vi "FGV_ARCH_EDITOR_records_display.vi"(4 "front_panel_reference":refnum<vi>, 6 "SQL_listbox_reference":refnum<vi>, 7 "options":T3, 8 "error_in":errorcluster, 10 "uneditable_columns":string[](array[string])=["ID", "CREATION_TIME", "CREATED_BY"], 11 "input":variant) -> (0 "error_out":errorcluster, 1 "all_info":T1, 2 "array_param_output":string[](array[string]), 3 "string_param_output":string)   [LabVIEW 2019]
uses:
  FGV_ARCH_EDITOR_records_display.ctl
  ARCH_EDITOR_all_info.ctl
  MAIN/SQL_record_states.ctl
  ini/typedef/CLIENT_all_config_info.ctl
  ini/typedef/CLIENT_main_ini_file.ctl
  queues/typedef/CLIENT_queue_refnums.ctl
  queues/typedef/SQL_EDITOR_queue_element.ctl
  MAIN/SQL_EDITOR/SQL_EDITOR_sequence_state.ctl
  queues/typedef/CLIENT_SCANNER_queue_element.ctl
  MAIN/SCANNER/SCANNER_sequence_state.ctl
  queues/typedef/CLIENT_REF_CHG_queue_element.ctl
  MAIN/reference_changed_connection/CLIENT_REF_CHG_sequence_state.ctl
  login/FGV_login.ctl
  <userlib>/_OpenG.lib/array/array.llb/Filter 1D Array (String)__ogtk.vi
  <userlib>/_OpenG.lib/array/array.llb/Delete Elements from 1D Array (I32)__ogtk.vi
  <vilib>/addons/database/_DB Variant To Data/Database Variant To Data.xnode
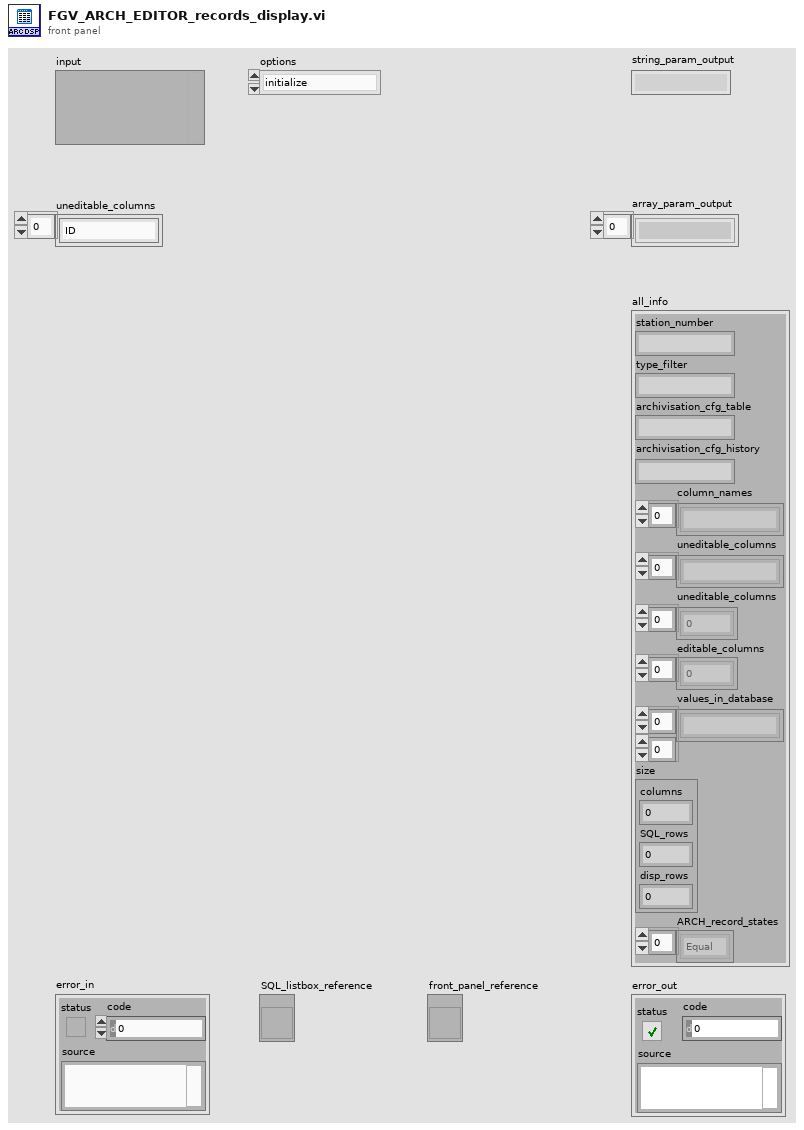
[diagram p1: front panel]
types:
  T1 = typedef "ARCH_EDITOR_all_info.ctl" = cluster{"station_number":string, "type_filter":string, "archivisation_cfg_table":string, "archivisation_cfg_history":string, "column_names":string[], "uneditable_columns":string[], "uneditable_columns":i32[], "editable_columns":i32[], "values_in_database":string[][], "size":cluster{"columns":i32, "SQL_rows":i32, "disp_rows":i32}, "ARCH_record_states":T2[]}
  T2 = typedef "SQL_record_states.ctl" = enum16{"Equal", "Added", "Edited", "Deleted"}
  T3 = typedef "FGV_ARCH_EDITOR_records_display.ctl" = enum16{"initialize", "set_arch_cfg_tables_names", "set_station_number", "set_type_filter", "set_headers", "set_records", "get_arch_cfg_table_name", "get_arch_cfg_hist_table_name", "get_station_number", "get_type_filter", "get_headers", "get_uneditable_columns", "get_all_info", "record_added?", "record_inserted?", "record_edited?", "record_updated?", "record_deleted?", "discard_changes"}
  T4 = typedef "CLIENT_all_config_info.ctl" = cluster{"main_ini_file":T5, "SQL Password":string, "queue_refnums":T6}
  T5 = typedef "CLIENT_main_ini_file.ctl" = cluster{"SQL Driver":string, "SQL Server":string, "SQL Database":string, "SQL UID":string, "Reference table":string, "Reference history":string, "Archivisation CFG table":string, "Archivisation CFG history":string, "User table":string, "User history":string, "logout timeout [ms]":i32, "records per page":i32, "default language":string, "REF CHG connection IP":string, "REF CHG remote port":i32, "REF CHG local port":i32, "SCANNER COM port":u16, "SCANNER Baud rate":u32, "SCANNER Data bits":u16, "SCANNER Pairity":enum16{"None", "Odd", "Even", "Mark", "Space"}, "SCANNER Stop bits":u16, "SCANNER Flow control":u16, "SCANNER Termination char":u8}
  T6 = typedef "CLIENT_queue_refnums.ctl" = cluster{"SQL_EDITOR_queue":refnum<queue>, "SCANNER_queue":refnum<queue>, "SCANNER_data":refnum<queue>, "CLIENT_REF_CHG_queue":refnum<queue>}
  T7 = typedef "FGV_login.ctl" = enum16{"initialize", "login", "logout", "get_login_info"}
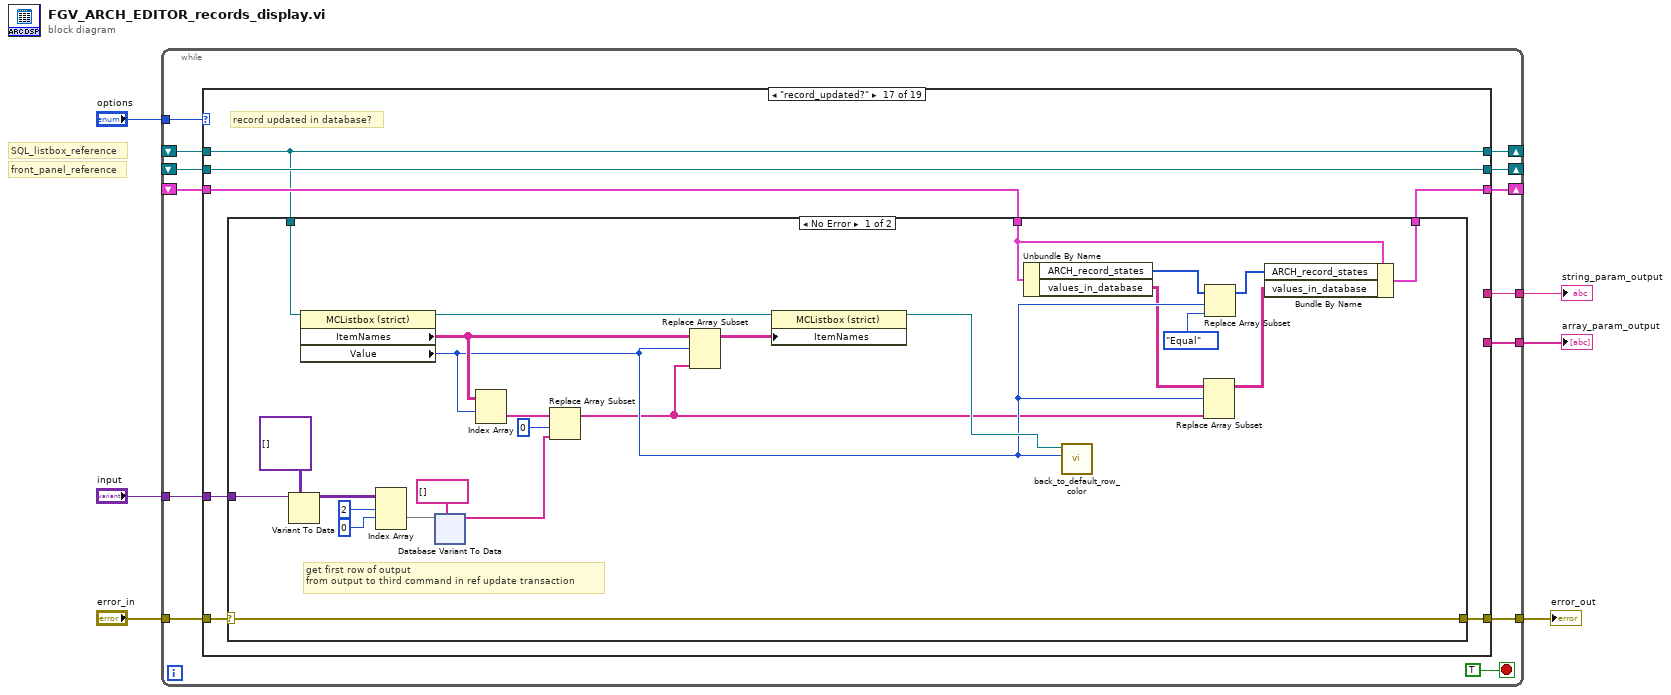
[diagram p0: block diagram]
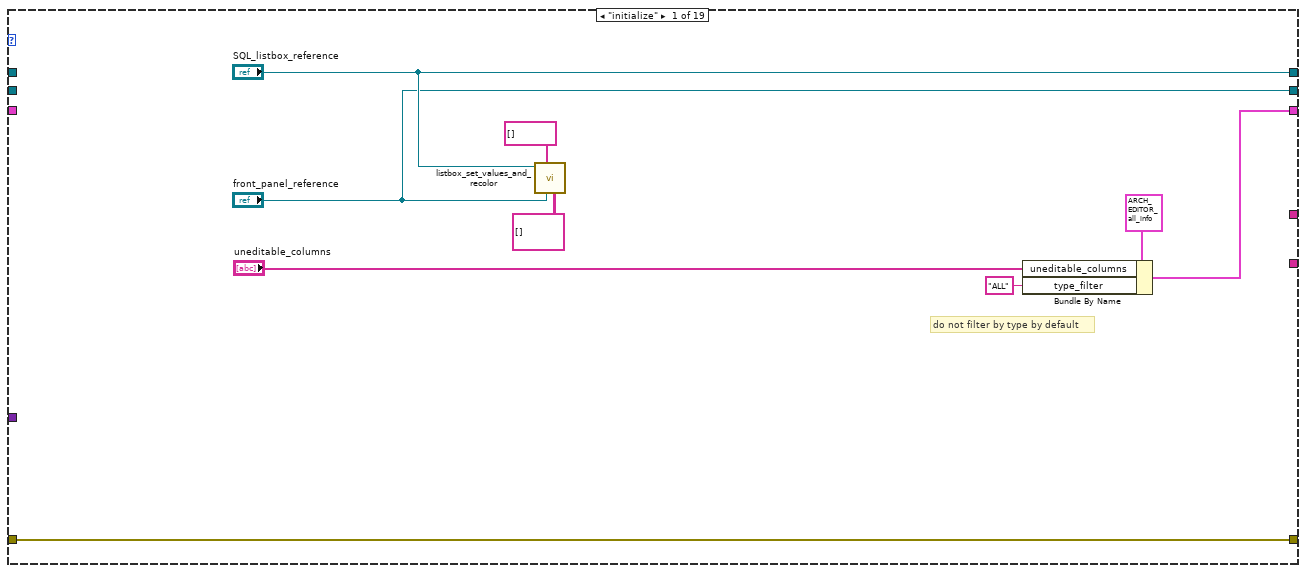
[diagram p2: hidden frame]
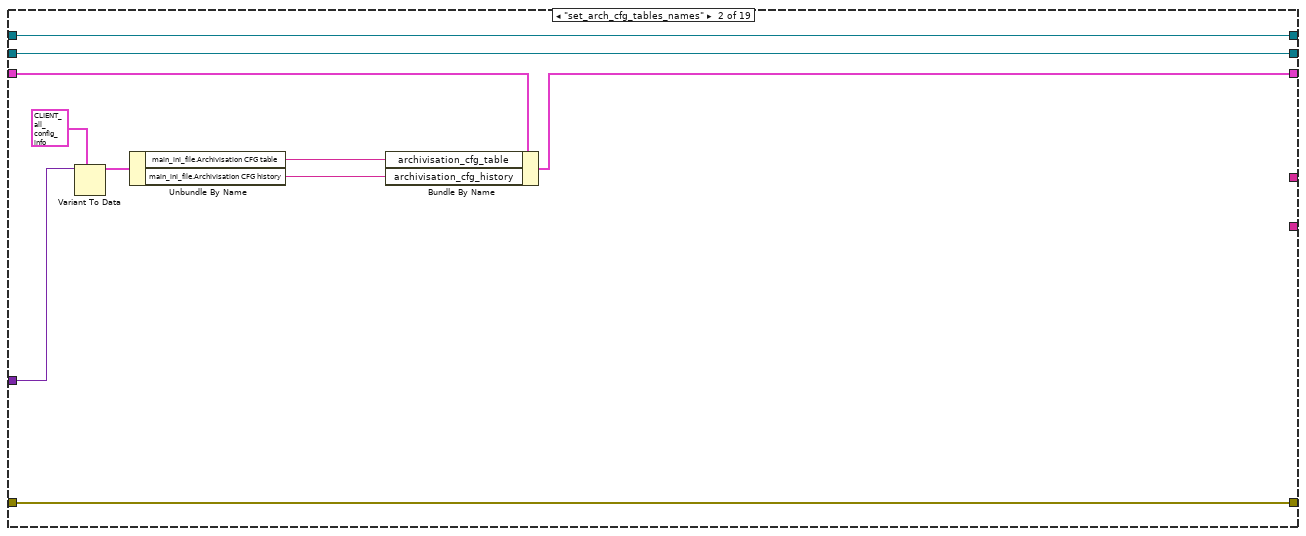
[diagram p3: hidden frame]
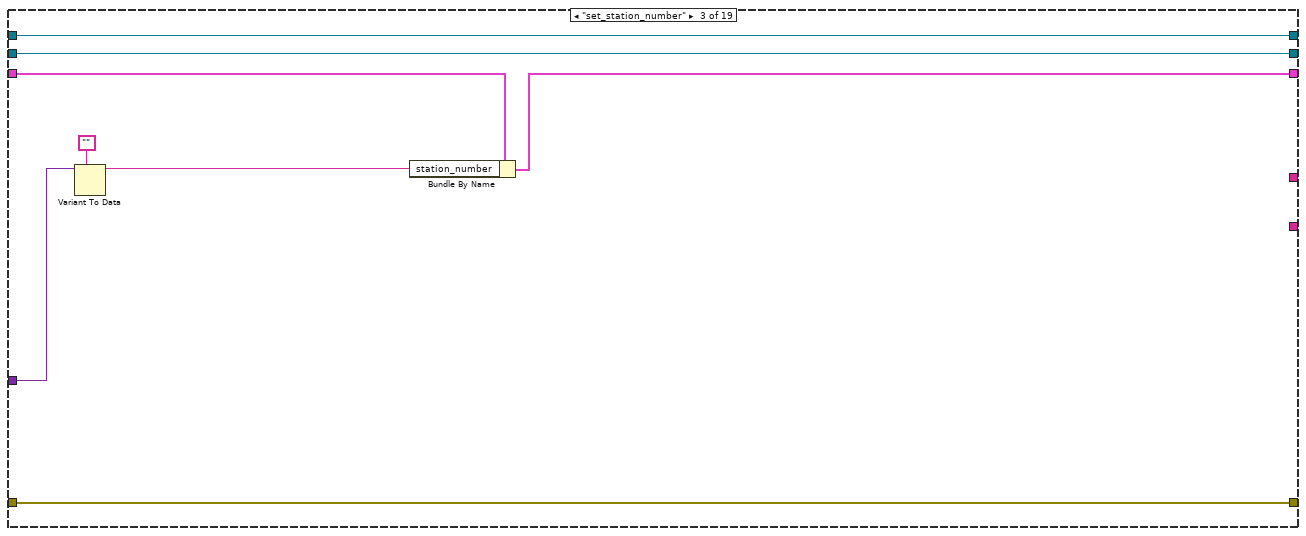
[diagram p4: hidden frame]
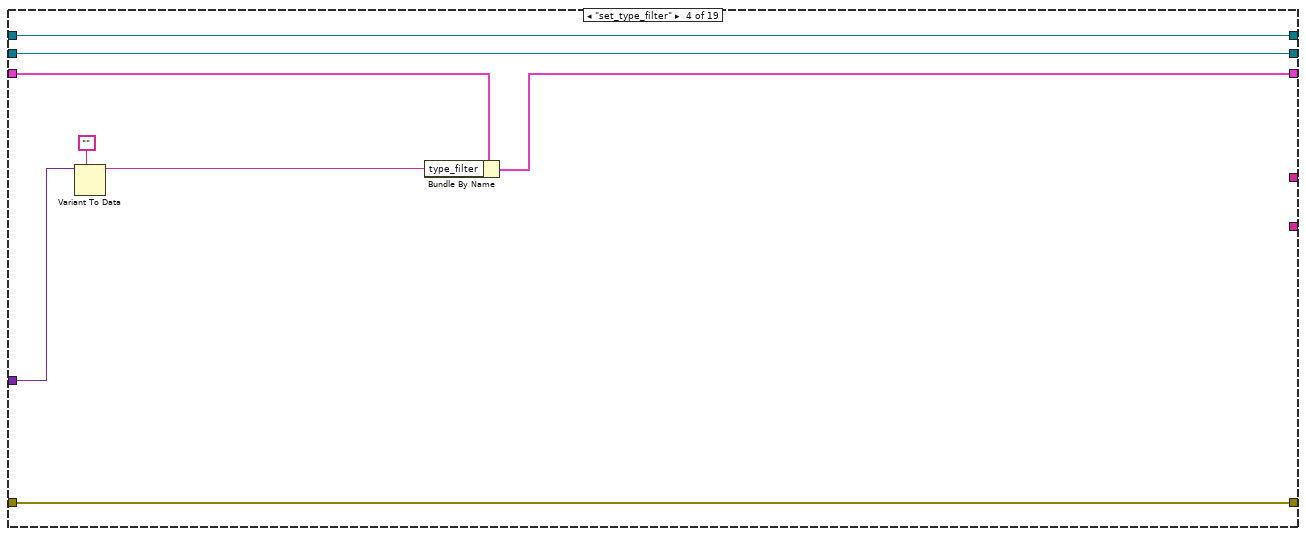
[diagram p5: hidden frame]
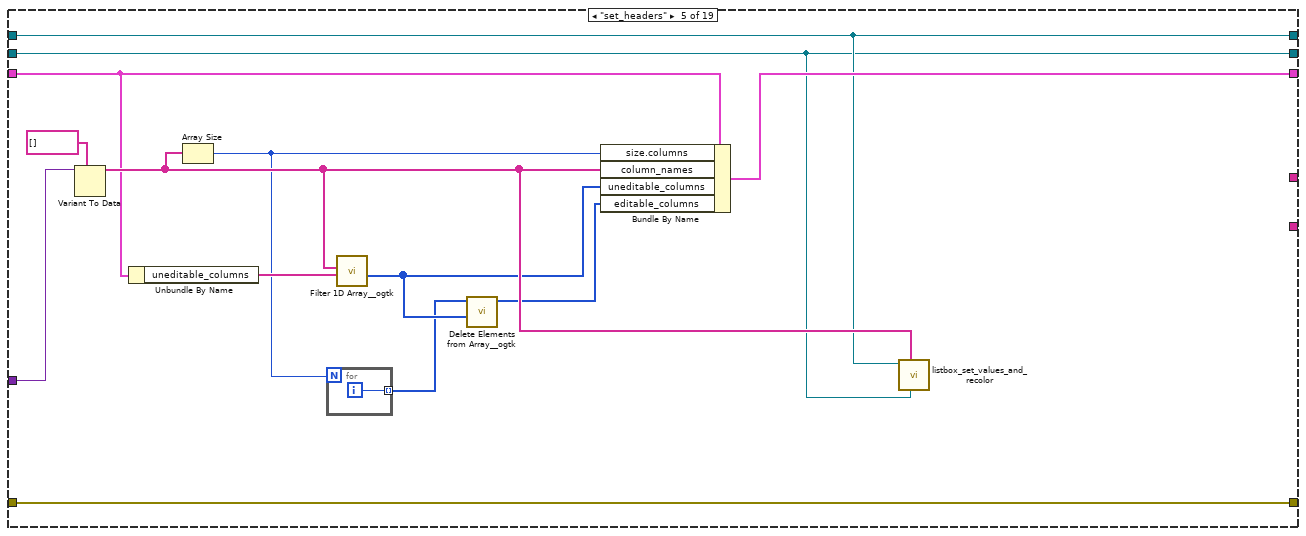
[diagram p6: hidden frame]
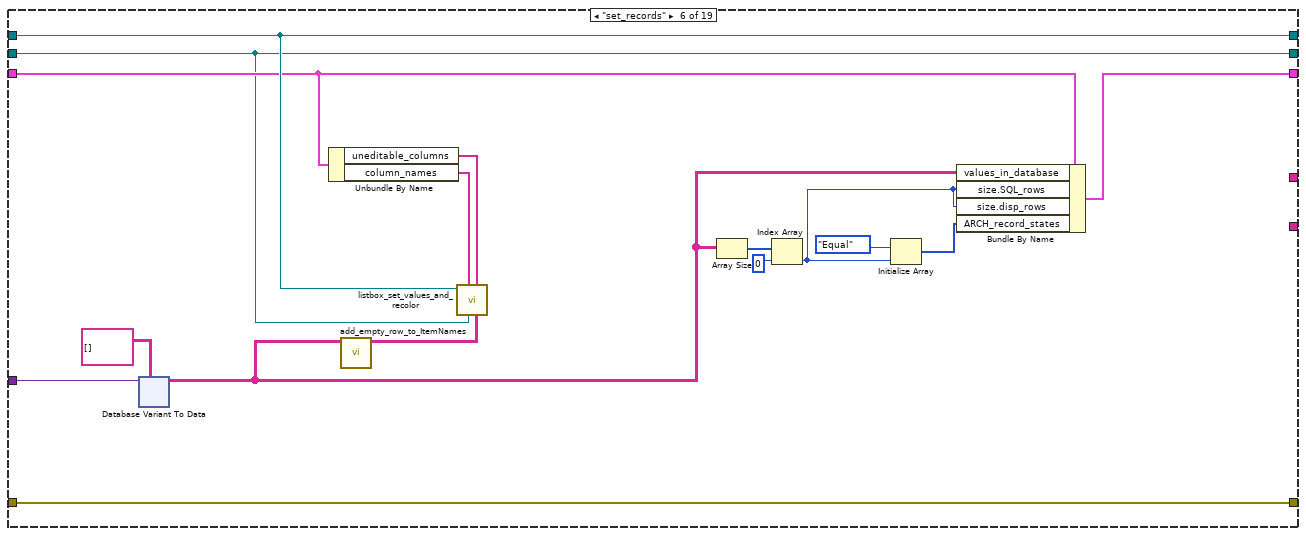
[diagram p7: hidden frame]
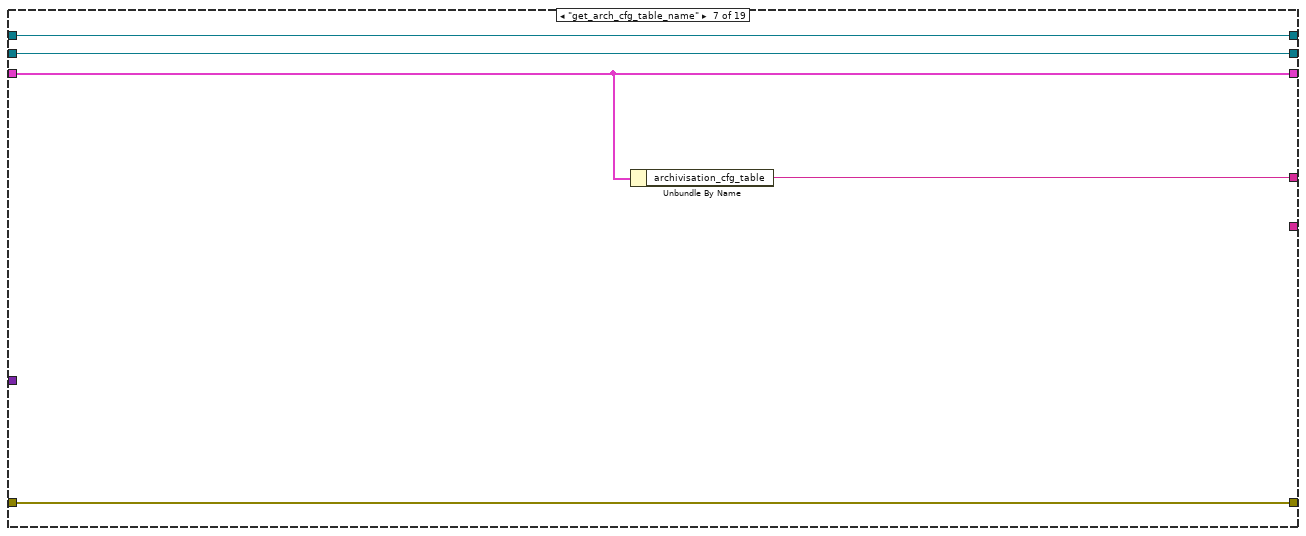
[diagram p8: hidden frame]
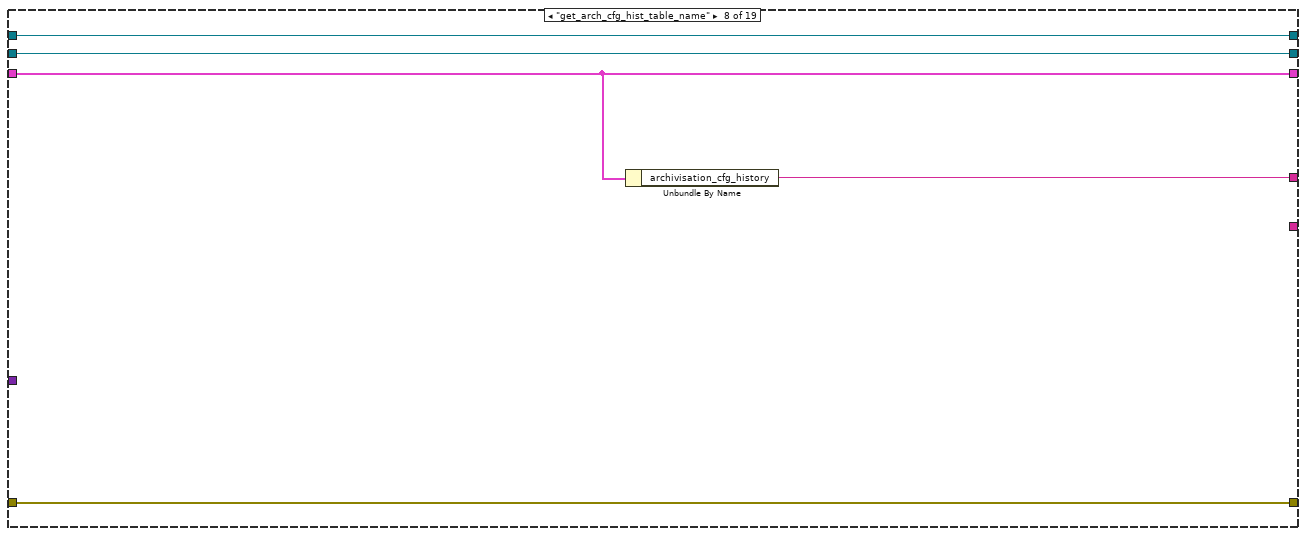
[diagram p9: hidden frame]
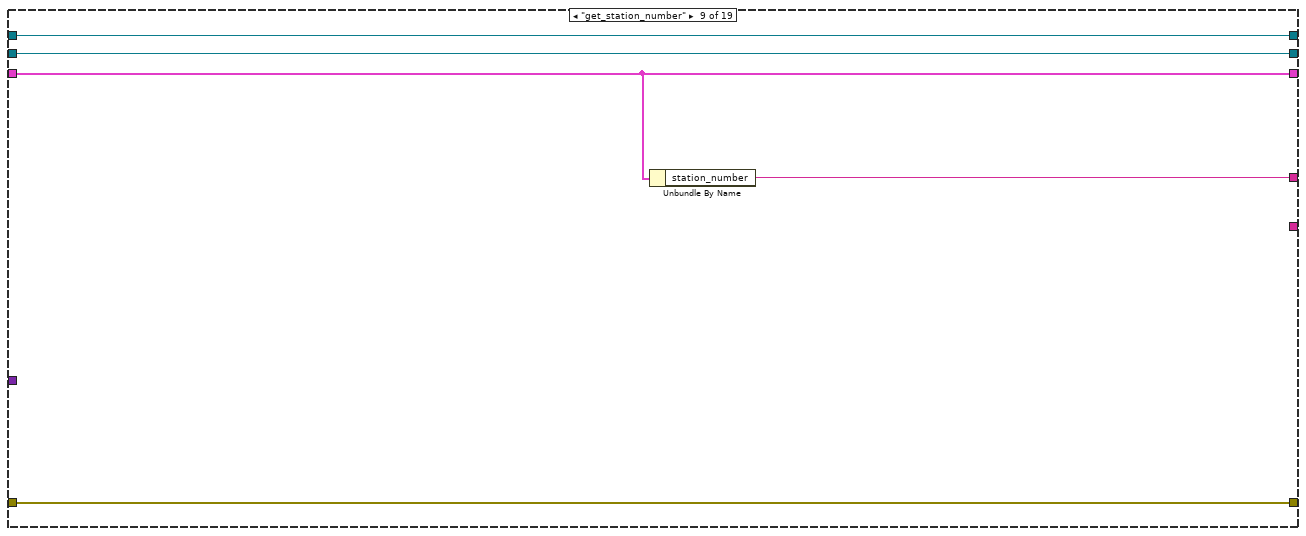
[diagram p10: hidden frame]
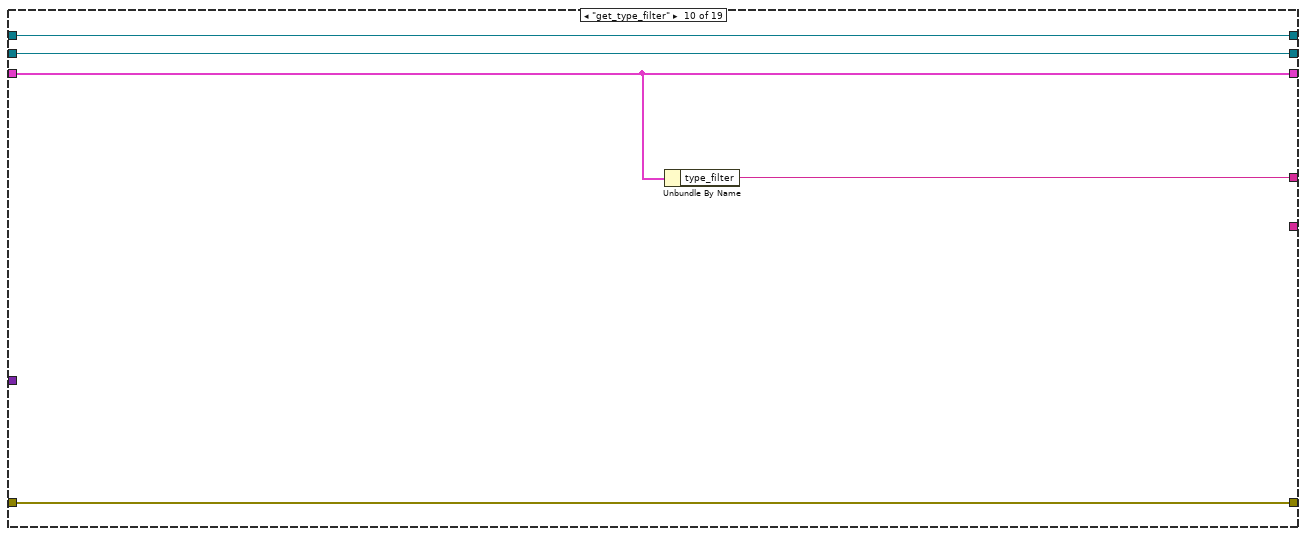
[diagram p11: hidden frame]
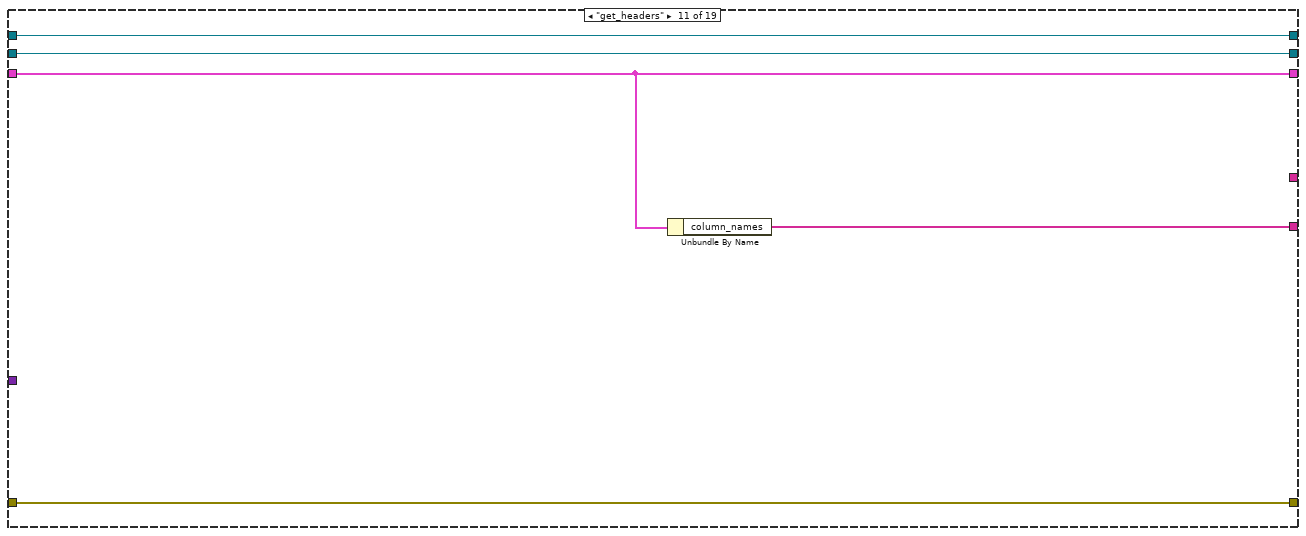
[diagram p12: hidden frame]
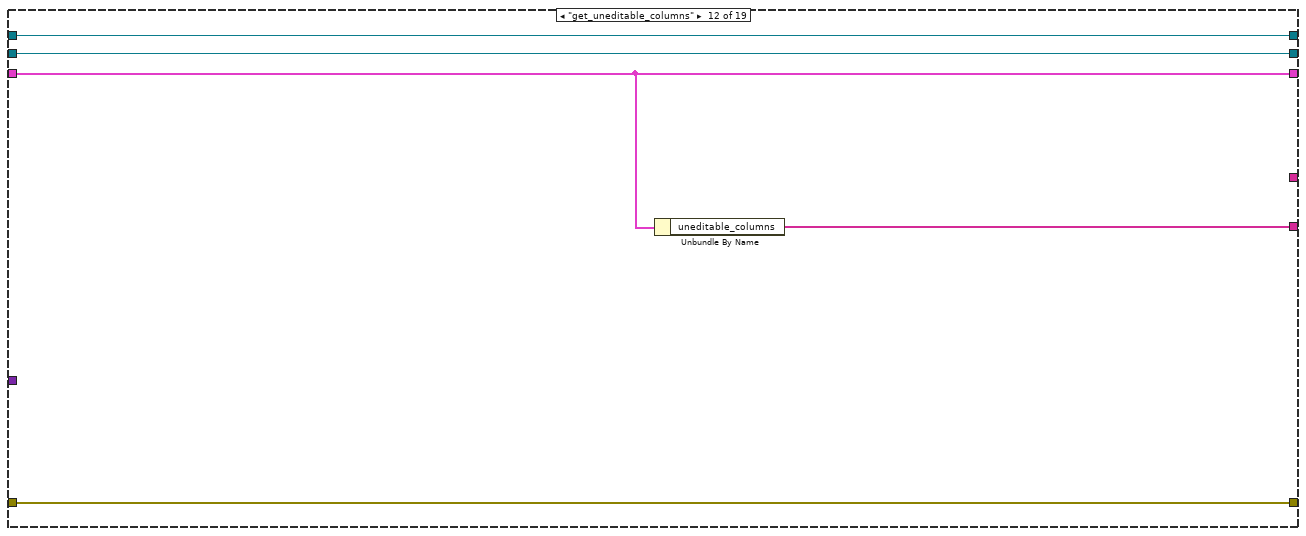
[diagram p13: hidden frame]
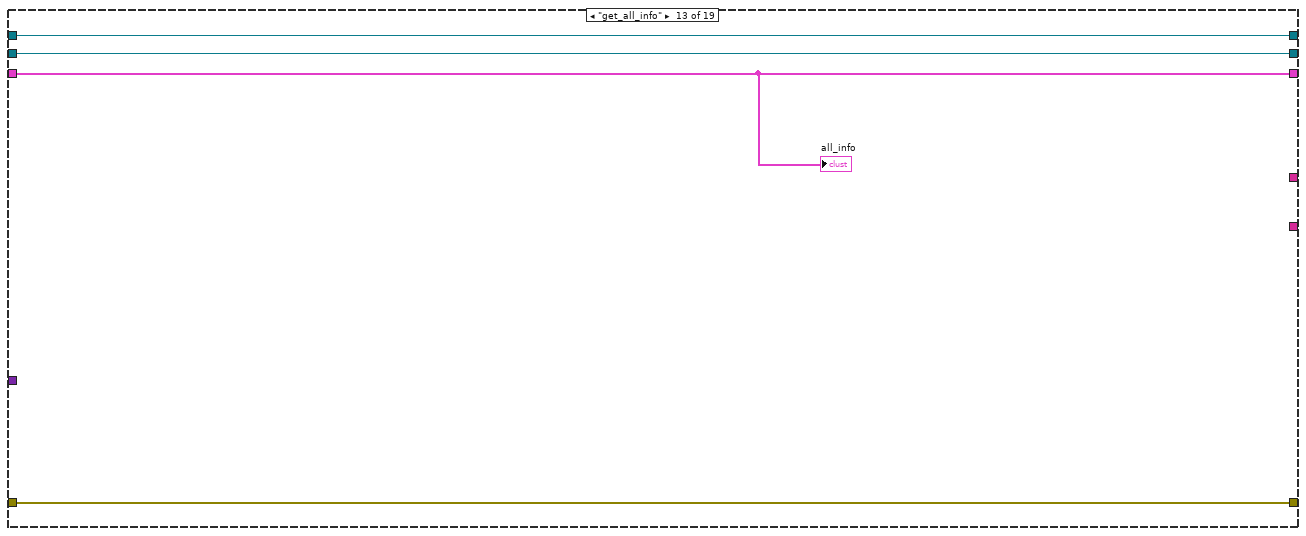
[diagram p14: hidden frame]
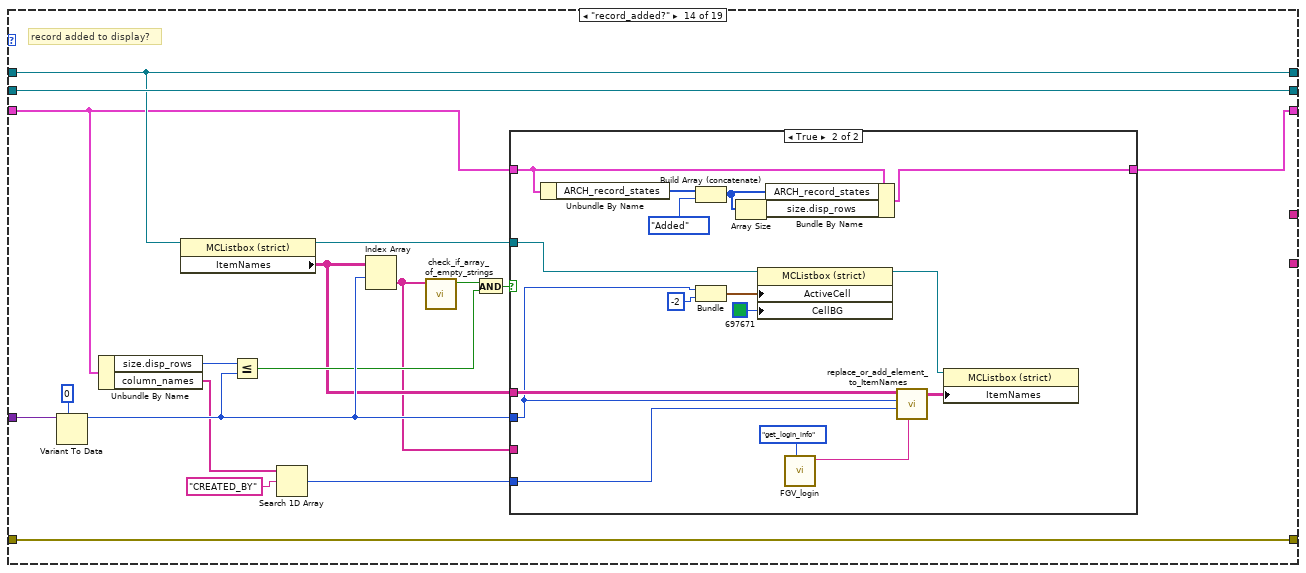
[diagram p15: hidden frame]
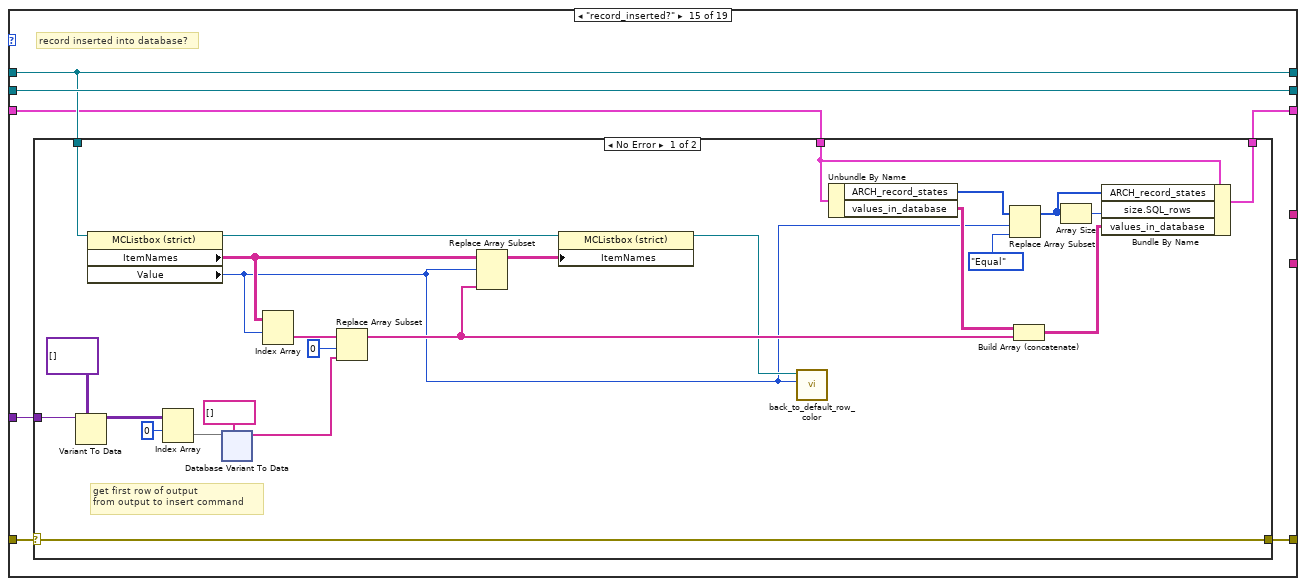
[diagram p17: hidden frame]
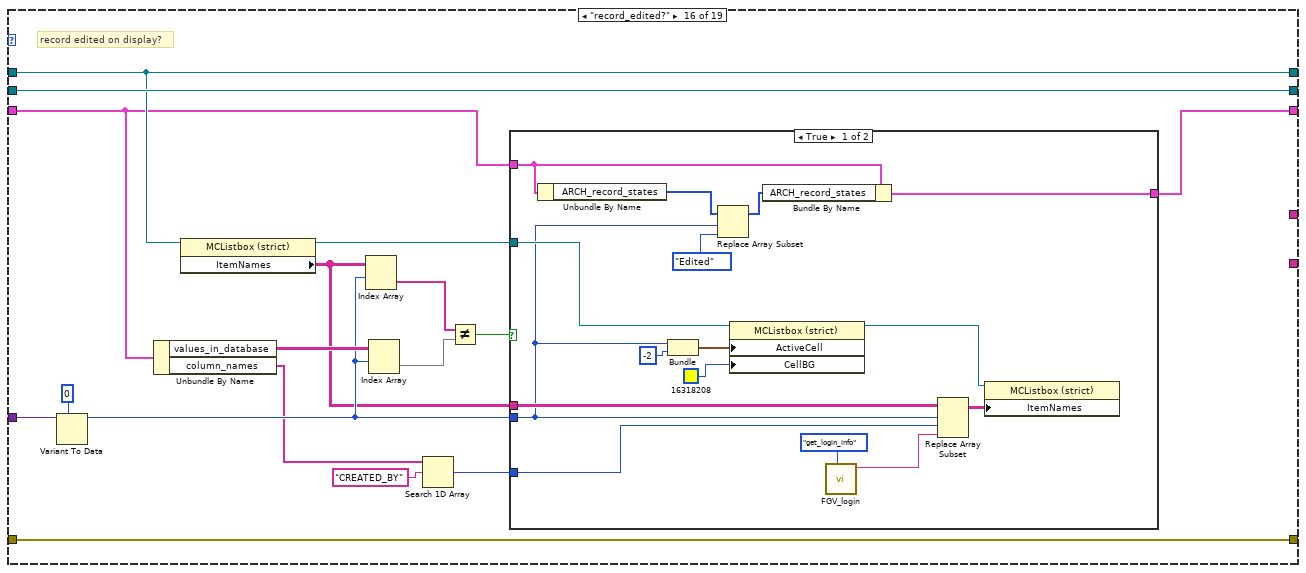
[diagram p19: hidden frame]
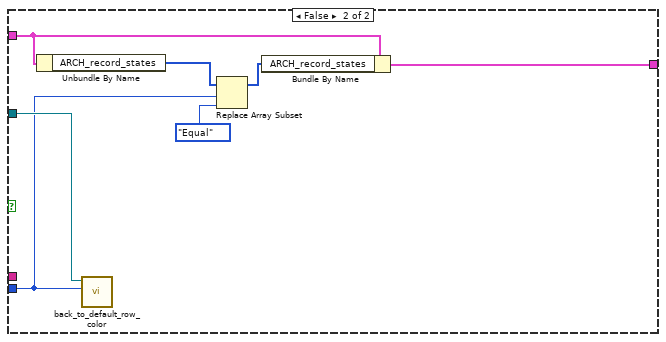
[diagram p20: hidden frame]
diagram:
  # "front_panel_reference"
  # "SQL_listbox_reference"
  n1 = while {
    tunnel: "options" -> [w18]
    tunnel: [w17] -> w6
    tunnel: "error_in" -> [w16]
    shift-right: [w15] -> _
    shift-left: _ -> [w14]
    tunnel: [w13] -> w3
    shift-right: [w12] -> _
    shift-left: _ -> [w11]
    tunnel: [w10] -> w2
    tunnel: "input" -> [w9]
    shift-right: [w8] -> _
    shift-left: _ -> [w7]
    stop <- TRUE stop-if-true
    n2 = case shown="\"record_updated?\"" w18 {
      tunnel: [w28 w38 w46 w54 w67 w82 w119 w124 w129 w134 w140 w145 w149 w168 w192 w275 w304 w372 w397] -> w17
      tunnel: w16 -> [w28 w38 w46 w54 w67 w82 w119 w124 w129 w134 w140 w145 w149 w168 w191 w275 w303 w373 w397]
      tunnel: [w24 w36 w44 w52 w57 w78 w121 w126 w131 w136 w141 w146 w150 w162 w188 w263 w300 w374 w398] -> w15
      tunnel: w14 -> [_ w37 w45 w53 w58 w79 w121 w126 w131 w136 w141 w146 w150 w161 w189 w264 w301 w375 w393]
      tunnel: [_ _ _ _ _ _ w120 w125 w130 w135 _ _ _ _ _ _ _ _ _] -> w13
      tunnel: ["SQL_listbox_reference" w35 w43 w51 w56 w81 w118 w123 w128 w133 w137 w144 w148 w164 w190 w270 w299 w377 w392] -> w12
      tunnel: w11 -> [_ w35 w43 w51 w56 w81 w118 w123 w128 w133 w137 w144 w148 w164 w190 w270 w299 w377 w392]
      tunnel: [_ _ _ _ _ _ _ _ _ _ w139 w143 _ _ _ _ _ _ _] -> w10
      tunnel: w9 -> [_ w34 w42 w50 w59 w83 _ _ _ _ _ _ _ w166 w187 w273 w302 _ _]
      tunnel: ["front_panel_reference" w33 w39 w47 w55 w71 w117 w122 w127 w132 w138 w142 w147 w167 w193 w274 w305 w378 w400] -> w8
      tunnel: w7 -> [_ w33 w39 w47 w55 w71 w117 w122 w127 w132 w138 w142 w147 w167 w193 w274 w305 w378 w400]
      frame "initialize" {
        # "do not filter by type by default"
        n3 = call "listbox_set_values_and_recolor.vi"("item_names"=string[][] [], "front_panel_reference"="front_panel_reference", "column_names"=string[] [], "multicolumn_listbox_reference_in"="SQL_listbox_reference") -> ()  [unwired: 6 in, 2 out]
        n4 = Bundle By Name(cluster=T1 {"station_number"="", "type_filter"="", "archivisation_cfg_table"="", "archivisation_cfg_history"="", "column_names"=[], "uneditable_columns"=[], "uneditable_columns"=[], "editable_columns"=[], "values_in_database"=[], "size"={"columns"=0, "SQL_rows"=0, "disp_rows"=0}, "ARCH_record_states"=[]} ("SQL_selection"), "uneditable_columns"="uneditable_columns", "type_filter"="ALL") -> (w24:T1)
      }
      frame "set_arch_cfg_tables_names" {
        n5 = Variant To Data(type=T4 {"main_ini_file"={"SQL Driver"="", "SQL Server"="", "SQL Database"="", "SQL UID"="", "Reference table"="", "Reference history"="", "Archivisation CFG table"="", "Archivisation CFG history"="", "User table"="", "User history"="", "logout timeout [ms]"=0, "records per page"=0, "default language"="", "REF CHG connection IP"="", "REF CHG remote port"=0, "REF CHG local port"=0, "SCANNER COM port"=0, "SCANNER Baud rate"=0, "SCANNER Data bits"=0, "SCANNER Pairity"=enum."None", "SCANNER Stop bits"=10, "SCANNER Flow control"=0, "SCANNER Termination char"=0}, "SQL Password"="", "queue_refnums"={"SQL_EDITOR_queue"=refnum, "SCANNER_queue"=refnum, "SCANNER_data"=refnum, "CLIENT_REF_CHG_queue"=refnum}} ("all_config_info"), Variant=w34) -> (data=w32:T4)  [unwired: 1 in, 1 out]
        n6 = Unbundle By Name(w32) -> ("main_ini_file.Archivisation CFG table"=w31:string, "main_ini_file.Archivisation CFG history"=w30:string)
        n7 = Bundle By Name(cluster=w37, "archivisation_cfg_table"=w31, "archivisation_cfg_history"=w30) -> (w36:T1)
      }
      frame "set_station_number" {
        n8 = Variant To Data(type="", Variant=w42) -> (data=w40:string)  [unwired: 1 in, 1 out]
        n9 = Bundle By Name(cluster=w45, "station_number"=w40) -> (w44:T1)
      }
      frame "set_type_filter" {
        n10 = Variant To Data(type="", Variant=w50) -> (data=w48:string)  [unwired: 1 in, 1 out]
        n11 = Bundle By Name(cluster=w53, "type_filter"=w48) -> (w52:T1)
      }
      frame "set_headers" {
        n12 = Variant To Data(type=string[] [], Variant=w59) -> (data=w65:string[])  [unwired: 1 in, 1 out]
        n13 = Unbundle By Name(w58) -> ("uneditable_columns"=w63:string[])
        n14 = Array Size(array=w65) -> (size(s)=w60:i32)
        n15 = for {
          N: w60 -> [_]
          tunnel: [w68] -> w62 mode=indexing
          i -> [w68]
        }
        n16 = call-poly <userlib>:"Filter 1D Array__ogtk.vi"("items to filter"=w63, "array"=w65) -> ("filtered item indices"=w64:i32[])  [unwired: 4 in, 1 out]
        n17 = call-poly <userlib>:"Delete Elements from Array__ogtk.vi"("indices"=w64, "array"=w62) -> ("array w/ subset deleted"=w61:i32[])  [unwired: 8 in, 1 out]
        n18 = Bundle By Name(cluster=w58, "size.columns"=w60, "column_names"=w65, "uneditable_columns"=w64, "editable_columns"=w61) -> (w57:T1)
        n19 = call "listbox_set_values_and_recolor.vi"("front_panel_reference"=w55, "column_names"=w65, "multicolumn_listbox_reference_in"=w56) -> ()  [unwired: 7 in, 2 out]
      }
      frame "set_records" {
        n20 = xnode "Database Variant To Data"("database variant"=w83, "type"=string[][] []) -> ("data"=w69:string[][])  [unwired: 1 in, 1 out]
        n21 = Unbundle By Name(w79) -> ("uneditable_columns"=w72:string[], "column_names"=w80:string[])
        n22 = call "add_empty_row_to_ItemNames.vi"("ItemNames_in"=w69) -> ("ItemNames_out"=w70:string[][])  [unwired: 10 in]
        n23 = call "listbox_set_values_and_recolor.vi"("item_names"=w70, "uneditable_columns"=w72, "front_panel_reference"=w71, "column_names"=w80, "multicolumn_listbox_reference_in"=w81) -> ()  [unwired: 5 in, 2 out]
        n24 = Array Size(array=w69) -> (size(s)=w77:i32[])
        n25 = Index Array(array=w77, index=0) -> (element=w74:i32)
        n26 = Initialize Array(SQL_record_states."Equal", w74) -> (w73:T2[])
        n27 = Bundle By Name(cluster=w79, "values_in_database"=w69, "size.SQL_rows"=w74, "size.disp_rows"=w74, "ARCH_record_states"=w73) -> (w78:T1)
      }
      frame "get_arch_cfg_table_name" {
        n28 = Unbundle By Name(w121) -> ("archivisation_cfg_table"=w120:string)
      }
      frame "get_arch_cfg_hist_table_name" {
        n29 = Unbundle By Name(w126) -> ("archivisation_cfg_history"=w125:string)
      }
      frame "get_station_number" {
        n30 = Unbundle By Name(w131) -> ("station_number"=w130:string)
      }
      frame "get_type_filter" {
        n31 = Unbundle By Name(w136) -> ("type_filter"=w135:string)
      }
      frame "get_headers" {
        n32 = Unbundle By Name(w141) -> ("column_names"=w139:string[])
      }
      frame "get_uneditable_columns" {
        n33 = Unbundle By Name(w146) -> ("uneditable_columns"=w143:string[])
      }
      frame "get_all_info" {
        "all_info" <- w150
      }
      frame "record_added?" {
        # "record added to display?"
        n34 = Variant To Data(type=0, Variant=w166) -> (data=w159:i32)  [unwired: 1 in, 1 out]
        n35 = Unbundle By Name(w161) -> ("size.disp_rows"=w160:i32, "column_names"=w156:string[])
        n36 = property class="MCListbox (strict)"(reference=w164) -> (reference out=w163:refnum<vi>, "ItemNames"=w157:string[][])  [unwired: 1 in, 1 out]
        n37 = Less Or Equal?(x=w160, y=w159) -> (x <= y?=w158:bool)
        n38 = Search 1D Array(1D array=w156, element="CREATED_BY") -> (index of element=w154:i32)  [unwired: 1 in]
        n39 = Index Array(array=w157, index (row)=w159) -> (element=w153:string[])  [unwired: 1 in]
        n40 = call "check_if_array_of_empty_strings.vi"("array"=w153) -> ("Not empty?"=w151:bool)  [unwired: 10 in]
        n41 = And(x=w151, y=w158) -> (x .and. y?=w152:bool)
        n42 = case shown="True" w152 {
          tunnel: w159 -> [_ w174]
          tunnel: w163 -> [_ w183]
          tunnel: w161 -> [w169 w181]
          tunnel: [w169 w182] -> w162
          tunnel: w157 -> [_ w175]
          tunnel: w153 -> [_ _]
          tunnel: w154 -> [_ w173]
          frame False {
          }
          frame True {
            n43 = Unbundle By Name(w181) -> ("ARCH_record_states"=w180:T2[])
            n44 = Build Array (concatenate)(w180, SQL_record_states."Added" ("new element/subarray")) -> (w178:T2[])
            n45 = Bundle(w174, -2) -> (w184:cluster{i32, i32})  [unwired: 1 in]
            n46 = Array Size(array=w178) -> (size(s)=w177:i32)
            n47 = property on="Property Node" class="MCListbox (strict)"(reference=w183, "ActiveCell"=w184, "CellBG"=u32 697671) -> (reference out=w172:refnum<vi>)  [unwired: 1 in, 1 out]
            n48 = Bundle By Name(cluster=w181, "ARCH_record_states"=w178, "size.disp_rows"=w177) -> (w182:T1)
            n49 = call "FGV_login.vi"("options"=FGV_login."get_login_info") -> ("username_out"=w170:string)  [unwired: 8 in, 2 out]
            n50 = call "replace_or_add_element_to_ItemNames.vi"("element"=w170, "column"=w173, "row"=w174, "ItemNames_in"=w175) -> ("ItemNames_out"=w176:string[][])  [unwired: 7 in]
            n51 = property class="MCListbox (strict)"(reference=w172, "ItemNames"=w176) -> ()  [unwired: 1 in, 2 out]
          }
        }
      }
      frame "record_inserted?" {
        # "record inserted into database?"
        n52 = case shown="No Error" w191 {
          selector: w191 -> [w194 w258]
          tunnel: w189 -> [w218 w257]
          tunnel: [w217 w257] -> w188
          tunnel: w187 -> [w200 _]
          tunnel: w190 -> [w199 _]
          tunnel: [w194 w258] -> w192
          frame No Error {
            # "get first row of output\nfrom output to insert command"
            n53 = Variant To Data(type=variant[][] [], Variant=w200) -> (data=w209:variant[][])  [unwired: 1 in, 1 out]
            n54 = property class="MCListbox (strict)"(reference=w199) -> (reference out=w203:refnum<vi>, "ItemNames"=w202:string[][], "Value"=w196:i32)  [unwired: 1 in, 1 out]
            n55 = Index Array(array=w209, index (row)=0) -> (element=w206:variant[])  [unwired: 1 in]
            n56 = xnode "Database Variant To Data"("database variant"=w206, "type"=string[] []) -> ("data"=w204:string[])  [unwired: 1 in, 1 out]
            n57 = Index Array(array=w202, index (row)=w196) -> (element=w208:string[])  [unwired: 1 in]
            n58 = Replace Array Subset(array=w208, new element=w204, index=0) -> (w198:string[])
            n59 = Replace Array Subset(array=w202, new element=w198, index (row)=w196) -> (w201:string[][])  [unwired: 1 in]
            n60 = property class="MCListbox (strict)"(reference=w203, "ItemNames"=w201) -> (reference out=w197:refnum<vi>)  [unwired: 1 in, 1 out]
            n61 = call "back_to_default_row_color.vi"("row"=w196, "listbox_reference"=w197) -> ()  [unwired: 9 in, 1 out]
            n62 = Unbundle By Name(w218) -> ("ARCH_record_states"=w215:T2[], "values_in_database"=w214:string[][])
            n63 = Replace Array Subset(array=w215, new element=SQL_record_states."Equal" ("new element/subarray"), index=w196) -> (w211:T2[])
            n64 = Build Array (concatenate)(w214, w198) -> (w213:string[][])
            n65 = Array Size(array=w211) -> (size(s)=w212:i32)
            n66 = Bundle By Name(cluster=w218, "ARCH_record_states"=w211, "size.SQL_rows"=w212, "values_in_database"=w213) -> (w217:T1)
          }
          frame Error {
          }
        }
      }
      frame "record_edited?" {
        # "record edited on display?"
        n67 = Variant To Data(type=0, Variant=w273) -> (data=w265:i32)  [unwired: 1 in, 1 out]
        n68 = Unbundle By Name(w264) -> ("values_in_database"=w271:string[][], "column_names"=w260:string[])
        n69 = property class="MCListbox (strict)"(reference=w270) -> (reference out=w266:refnum<vi>, "ItemNames"=w262:string[][])  [unwired: 1 in, 1 out]
        n70 = Index Array(array=w262, index (row)=w265) -> (element=w269:string[])  [unwired: 1 in]
        n71 = Index Array(array=w271, index (row)=w265) -> (element=w268:string[])  [unwired: 1 in]
        n72 = Search 1D Array(1D array=w260, element="CREATED_BY") -> (index of element=w259:i32)  [unwired: 1 in]
        n73 = Not Equal?(x=w269, y=w268) -> (x != y?=w267:bool)
        n74 = case shown="True" w267 {
          tunnel: w265 -> [w277 w292]
          tunnel: w266 -> [w289 w293]
          tunnel: w264 -> [w285 w296]
          tunnel: [w283 w294] -> w263
          tunnel: w262 -> [w278 _]
          tunnel: w259 -> [w276 _]
          frame True {
            n75 = Unbundle By Name(w285) -> ("ARCH_record_states"=w286:T2[])
            n76 = Bundle(w277, -2) -> (w290:cluster{i32, i32})  [unwired: 1 in]
            n77 = Replace Array Subset(array=w286, new element=SQL_record_states."Edited" ("new element/subarray"), index=w277) -> (w284:T2[])
            n78 = property on="Property Node" class="MCListbox (strict)"(reference=w289, "ActiveCell"=w290, "CellBG"=u32 16318208) -> (reference out=w279:refnum<vi>)  [unwired: 1 in, 1 out]
            n79 = Bundle By Name(cluster=w285, "ARCH_record_states"=w284) -> (w283:T1)
            n80 = call "FGV_login.vi"("options"=FGV_login."get_login_info") -> ("username_out"=w280:string)  [unwired: 8 in, 2 out]
            n81 = Replace Array Subset(array=w278, new element=w280, index (row)=w277, index (col)=w276) -> (w282:string[][])
            n82 = property class="MCListbox (strict)"(reference=w279, "ItemNames"=w282) -> ()  [unwired: 1 in, 2 out]
          }
          frame False {
            n83 = Unbundle By Name(w296) -> ("ARCH_record_states"=w297:T2[])
            n84 = call "back_to_default_row_color.vi"("row"=w292, "listbox_reference"=w293) -> ()  [unwired: 9 in, 1 out]
            n85 = Replace Array Subset(array=w297, new element=SQL_record_states."Equal" ("new element/subarray"), index=w292) -> (w295:T2[])
            n86 = Bundle By Name(cluster=w296, "ARCH_record_states"=w295) -> (w294:T1)
          }
        }
      }
      frame "record_updated?" {
        # "record updated in database?"
        n87 = case shown="No Error" w303 {
          selector: w303 -> [w307 w369]
          tunnel: w299 -> [w330 _]
          tunnel: w301 -> [w329 w370]
          tunnel: [w328 w370] -> w300
          tunnel: w302 -> [w327 _]
          tunnel: [w307 w369] -> w304
          frame No Error {
            # "get first row of output\nfrom output to third command in ref update transaction"
            n88 = Variant To Data(type=variant[][][] [], Variant=w327) -> (data=w325:variant[][][])  [unwired: 1 in, 1 out]
            n89 = property class="MCListbox (strict)"(reference=w330) -> (reference out=w317:refnum<vi>, "ItemNames"=w315:string[][], "Value"=w314:i32)  [unwired: 1 in, 1 out]
            n90 = Index Array(array=w325, index (dim 0)=2 ("index (page)"), index (dim 1)=0 ("disabled index (row)")) -> (element=w320:variant[])  [unwired: 1 in]
            n91 = xnode "Database Variant To Data"("database variant"=w320, "type"=string[] []) -> ("data"=w318:string[])  [unwired: 1 in, 1 out]
            n92 = Index Array(array=w315, index (row)=w314) -> (element=w322:string[])  [unwired: 1 in]
            n93 = Replace Array Subset(array=w322, new element=w318, index=0) -> (w313:string[])
            n94 = Replace Array Subset(array=w315, new element=w313, index (row)=w314) -> (w306:string[][])  [unwired: 1 in]
            n95 = property class="MCListbox (strict)"(reference=w317, "ItemNames"=w306) -> (reference out=w316:refnum<vi>)  [unwired: 1 in, 1 out]
            n96 = Unbundle By Name(w329) -> ("ARCH_record_states"=w311:T2[], "values_in_database"=w308:string[][])
            n97 = call "back_to_default_row_color.vi"("row"=w314, "listbox_reference"=w316) -> ()  [unwired: 9 in, 1 out]
            n98 = Replace Array Subset(array=w308, new element=w313, index (row)=w314) -> (w309:string[][])  [unwired: 1 in]
            n99 = Replace Array Subset(array=w311, new element=SQL_record_states."Equal" ("new element/subarray"), index=w314) -> (w310:T2[])
            n100 = Bundle By Name(cluster=w329, "ARCH_record_states"=w310, "values_in_database"=w309) -> (w328:T1)
          }
          frame Error {
          }
        }
      }
      frame "record_deleted?" {
        # "record deleted from database?"
        n101 = property class="MCListbox (strict)"(reference=w377) -> (reference out=w376:refnum<vi>, "Value"=w371:i32)  [unwired: 1 in, 1 out]
        n102 = case shown="No Error" w373 {
          selector: w373 -> [w380 w381]
          tunnel: w376 -> [_ w389]
          tunnel: w375 -> [w379 w385]
          tunnel: [w379 w383] -> w374
          tunnel: [w380 w381] -> w372
          tunnel: w371 -> [_ w382]
          frame Error {
          }
          frame No Error {
            n103 = Unbundle By Name(w385) -> ("ARCH_record_states"=w386:T2[])
            n104 = Bundle("Value"=w382, -2) -> (w390:cluster{"Value":i32, i32})  [unwired: 1 in]
            n105 = Replace Array Subset(array=w386, new element=SQL_record_states."Deleted" ("new element/subarray"), index=w382) -> (w384:T2[])
            n106 = property on="Property Node" class="MCListbox (strict)"(reference=w389, "ActiveCell"=w390, "CellBG"=u32 16711763) -> ()  [unwired: 1 in, 2 out]
            n107 = Bundle By Name(cluster=w385, "ARCH_record_states"=w384) -> (w383:T1)
          }
        }
      }
      frame "discard_changes" {
        # "discard changes on display"
        n108 = property class="MCListbox (strict)"(reference=w392) -> (reference out=w399:refnum<vi>, "Value"=w395:i32)  [unwired: 1 in, 1 out]
        n109 = Unbundle By Name(w393) -> ("ARCH_record_states"=w396:T2[])
        n110 = Index Array(array=w396, index=w395) -> (element=w394:T2)
        n111 = case shown="\"Edited\"" w394 {
          tunnel: w399 -> [_ w415 w421]
          tunnel: w393 -> [w401 w414 w430]
          tunnel: [w401 w413 w429] -> w398
          tunnel: w395 -> [_ w405 w420]
          tunnel: w393 -> [_ w410 w428]
          tunnel: w392 -> [_ w408 w426]
          frame Default {
          }
          frame "Edited" {
            n112 = Unbundle By Name(w410) -> ("values_in_database"=w406:string[][], "ARCH_record_states"=w409:T2[])
            n113 = property class="MCListbox (strict)"(reference=w408) -> (reference out=w403:refnum<vi>, "ItemNames"=w407:string[][])  [unwired: 1 in, 1 out]
            n114 = call "back_to_default_row_color.vi"("row"=w405, "listbox_reference"=w415) -> ()  [unwired: 9 in, 1 out]
            n115 = Index Array(array=w406, index (row)=w405) -> (element=w404:string[])  [unwired: 1 in]
            n116 = Replace Array Subset(array=w409, new element=SQL_record_states."Equal" ("new element/subarray"), index=w405) -> (w411:T2[])
            n117 = Replace Array Subset(array=w407, new element=w404, index (row)=w405) -> (w402:string[][])  [unwired: 1 in]
            n118 = property class="MCListbox (strict)"(reference=w403, "ItemNames"=w402) -> ()  [unwired: 1 in, 2 out]
            n119 = Bundle By Name(cluster=w414, "ARCH_record_states"=w411) -> (w413:T1)
          }
          frame "Added" {
            n120 = Unbundle By Name(w428) -> ("ARCH_record_states"=w427:T2[])
            n121 = property class="MCListbox (strict)"(reference=w426) -> (reference out=w416:refnum<vi>, "ItemNames"=w425:string[][])  [unwired: 1 in, 1 out]
            n122 = Bundle("Value"=w420, -2) -> (w424:cluster{"Value":i32, i32})  [unwired: 1 in]
            n123 = property on="Property Node" class="MCListbox (strict)"(reference=w421, "ActiveCell"=w424, "CellBG"=u32 16448250) -> ()  [unwired: 1 in, 2 out]
            n124 = Delete From Array(array=w427, index=w420) -> (array with subset deleted=w418:T2[])  [unwired: 1 in, 1 out]
            n125 = Delete From Array(array=w425, index (row)=w420) -> (array with subset deleted=w417:string[][])  [unwired: 2 in, 1 out]
            n126 = Array Size(array=w418) -> (size(s)=w419:i32)
            n127 = call "add_empty_row_to_ItemNames.vi"("multicolumn_listbox_reference_in"=w416, "ItemNames_in"=w417) -> ()  [unwired: 9 in, 1 out]
            n128 = Bundle By Name(cluster=w430, "size.disp_rows"=w419, "ARCH_record_states"=w418) -> (w429:T1)
          }
        }
      }
    }
  }
  "error_out" <- w6
  "string_param_output" <- w3
  "array_param_output" <- w2
